vi "testCmdLineParser.vi"(8 "error in (no error)":errorcluster) -> (0 "error out":errorcluster)   [LabVIEW 2018]
uses:
  <vilib>/addons/_JKI Toolkits/Caraya/classes/Assert/Assert False.vi
  <vilib>/addons/_JKI Toolkits/Caraya/classes/Assert/Assert True.vi
  <vilib>/addons/_JKI Toolkits/Caraya/classes/Test/Test.lvclass
  <vilib>/addons/_JKI Toolkits/Caraya/classes/Assert/Assert.lvclass
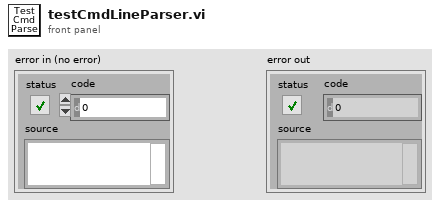
[diagram p1: front panel]
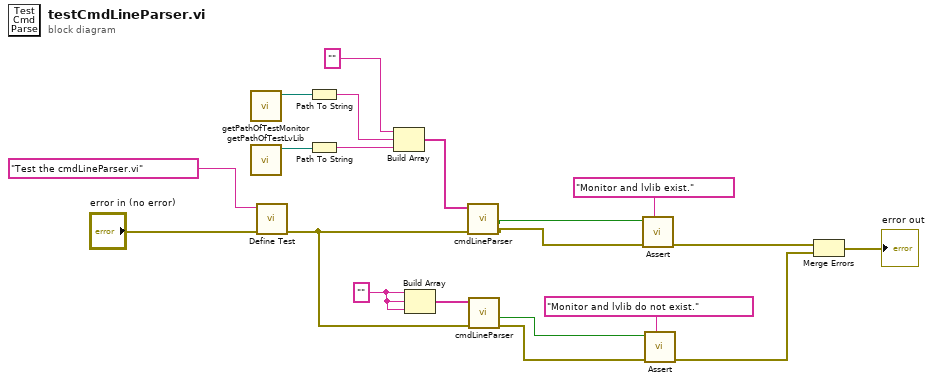
[diagram p0: block diagram]
diagram:
  w12 = ""
  n1 = call "getPathOfTestMonitor.vi"() -> ("testMonitorPath"=w14:path)  [unwired: 11 in]
  n2 = call "getPathOfTestLvLib.vi"() -> ("testLvLibPath"=w15:path)  [unwired: 11 in]
  n3 = call <vilib>:"Define Test.vi"("error in (no error)"="error in (no error)", "Label (VI Title)"="Test the cmdLineParser.vi") -> ("error out"=w10:errorcluster)  [unwired: 9 in]
  n4 = Path To String(path=w14) -> (string=w17:string)
  n5 = Path To String(path=w15) -> (string=w16:string)
  n6 = Build Array("", w17, w16) -> (w13:string[])
  n7 = Build Array(w12, w12, w12) -> (w11:string[])
  n8 = call "cmdLineParser.vi"("error in (no error)"=w10, "cmdLineArgs"=w13) -> ("error out"=w3:errorcluster, "filesExist"=w4:bool)  [unwired: 6 in, 2 out]
  n9 = call "cmdLineParser.vi"("error in (no error)"=w10, "cmdLineArgs"=w11) -> ("error out"=w2:errorcluster, "filesExist"=w1:bool)  [unwired: 6 in, 2 out]
  n10 = call-poly <vilib>:"Assert.vi"("Label"="Monitor and lvlib exist.", "error in (no error)"=w3, "True?"=w4) -> ("error out"=w7:errorcluster)  [unwired: 8 in]
  n11 = call-poly <vilib>:"Assert.vi"("Label"="Monitor and lvlib do not exist.", "error in (no error)"=w2, "False?"=w1) -> ("error out"=w6:errorcluster)  [unwired: 8 in]
  n12 = Merge Errors(w7, w6) -> (→"error out":errorcluster)
